vi "Measuring Complete Example (B).vi"() -> ()   [LabVIEW 2011]
uses:
  C:/Program Files/Metrohm Autolab/Autolab SDK 1.10/EcoChemie.Autolab.Sdk.dll
  EcoChemie.Autolab.Sdk.dll
panel:
  in  "Stop":bool
  out "PotentialApplied":dbl
  in  "Abort":bool
  in  "fileName":string
  out "IsMeasuring":bool
  in  "Save":bool
  in  "start measure":bool
  out "XY Graph":cluster{"Y":dbl[], "Y":dbl[]}[](graph)
  out "X: WE(1).Potential":dbl
  out "Y: WE(1).Current":dbl
  out "error out":errorcluster
  out "IsConnected":bool
  out "Y: EI_0.CalcCurrent":dbl[](array[numeric])
  out "X: SetpointApplied":dbl[](array[numeric])
  out "XY Graph 2":cluster{"Values":dbl[], "Values":dbl[]}(graph)
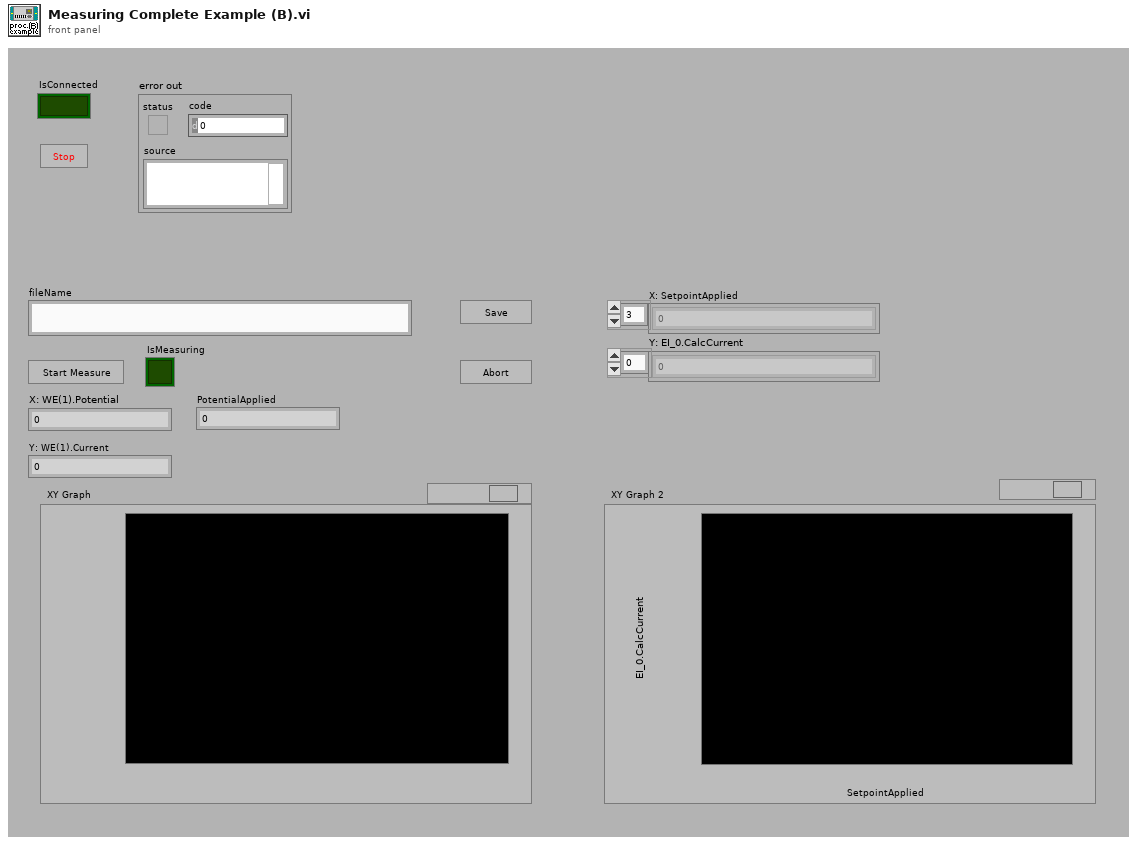
[diagram p1: front panel]
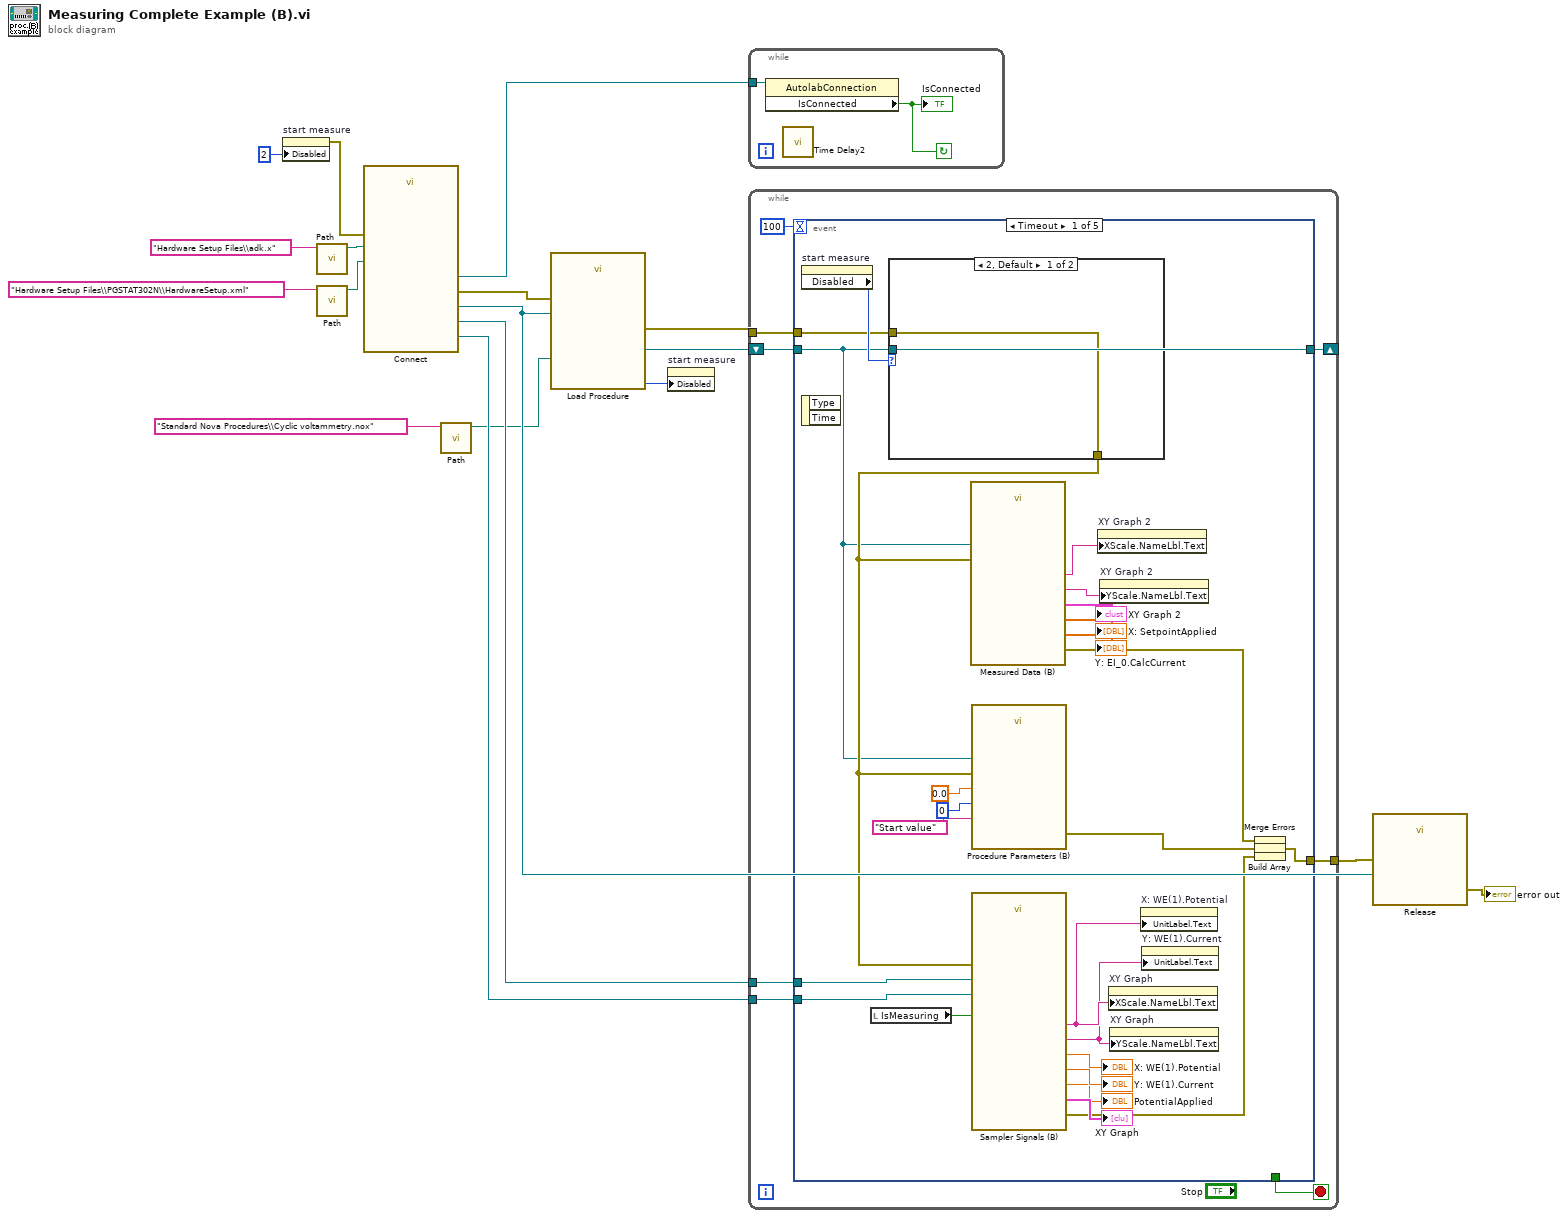
[diagram p0: block diagram]
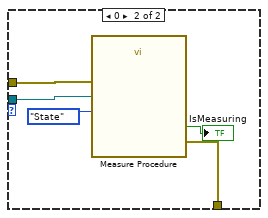
[diagram p2: hidden frame]
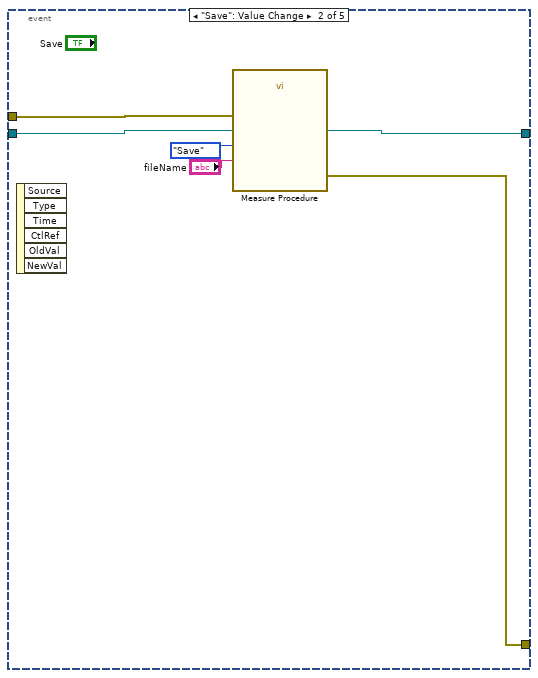
[diagram p3: hidden frame]
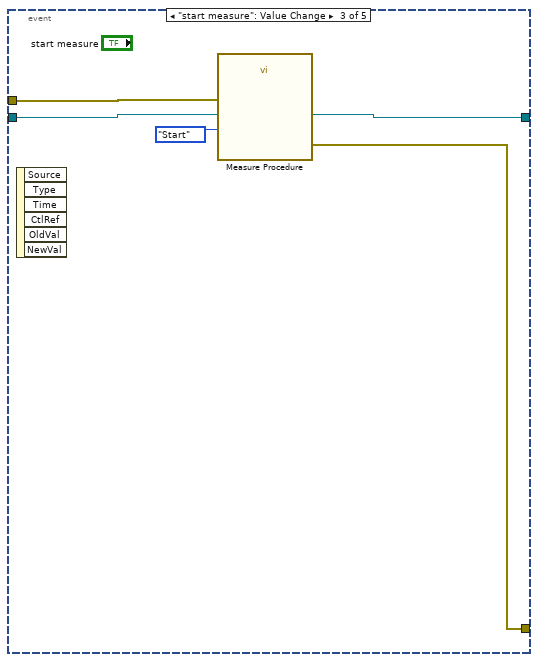
[diagram p4: hidden frame]
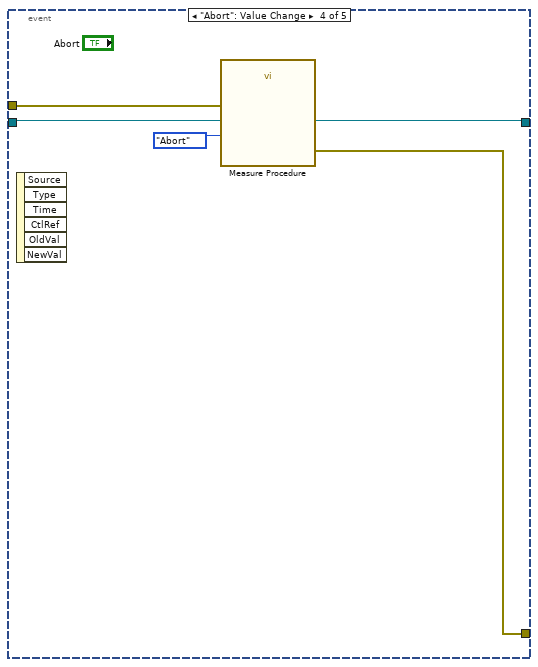
[diagram p5: hidden frame]
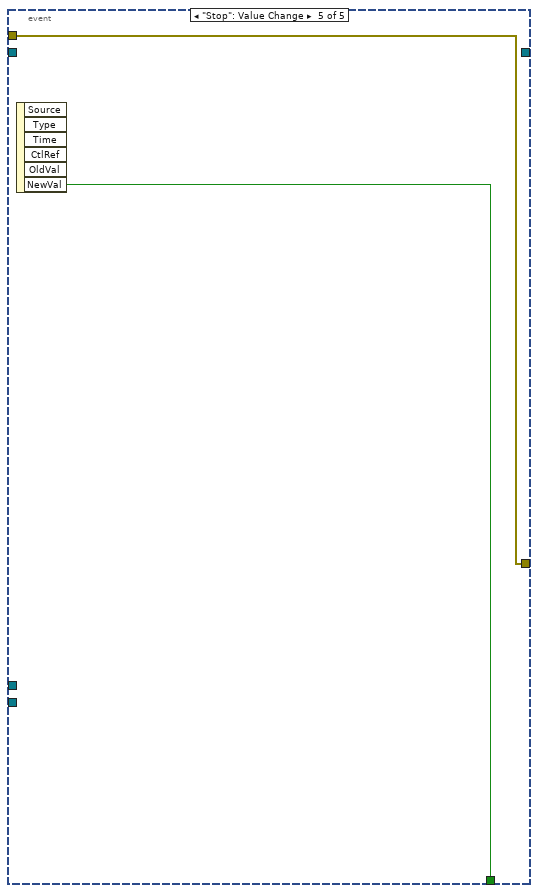
[diagram p6: hidden frame]
diagram:
  n1 = property on="start measure" class="Bool"("Disabled"=u8 2) -> (error out=w2:errorcluster)  [unwired: 2 in, 1 out]
  n2 = call "Path.vi"("name or relative path"="Hardware Setup Files\\adk.x") -> ("appended path"=w14:path)  [unwired: 10 in]
  n3 = call "Path.vi"("name or relative path"="Hardware Setup Files\\PGSTAT302N\\HardwareSetup.xml") -> ("appended path"=w11:path)  [unwired: 10 in]
  n4 = call "Connect.vi"("Embedded Exe File"=w14, "Hardware Setup File"=w11, "error in (no error)"=w2) -> ("Sampler"=w16:refnum<k24>, "AutolabConnection"=w17:refnum<k24>, "instrument"=w7:refnum<k24>, "Ei"=w15:refnum<k24>, "error out"=w8:errorcluster)  [unwired: 5 in, 3 out]
  n5 = call "Path.vi"("name or relative path"="Standard Nova Procedures\\Cyclic voltammetry.nox") -> ("appended path"=w4:path)  [unwired: 10 in]
  n6 = call "Load Procedure.vi"("error in (no error)"=w8, "Procedure"=w4, "Instrument"=w7) -> ("error out"=w6:errorcluster, "Numeric"=w3:i32, "LoadProcedure"=w5:refnum<k24>)  [unwired: 5 in, 1 out]
  n7 = property on="start measure" class="Bool"("Disabled"=w3) -> ()  [unwired: 2 in, 2 out]
  n8 = while {
    tunnel: w17 -> [w19]
    stop <- w20 continue-if-true
    n9 = property class="AutolabConnection"(reference=w19) -> ("IsConnected"=w20:bool)  [unwired: 1 in, 2 out]
    "IsConnected" <- w20
    n10 = call "Time Delay2"() -> ()  [unwired: 11 in, 1 out]
  }
  n11 = while {
    tunnel: w16 -> [w28]
    tunnel: w15 -> [w27]
    shift-right: [w25] -> _
    shift-left: w5 -> [w26]
    tunnel: w6 -> [w24]
    tunnel: [w22] -> w9
    stop <- w21 stop-if-true
    n12 = event shown="[0] Timeout" {
      selector: _ -> [_ _ _ _ _]
      dyn-events: _ -> [_ _ _ _ _]
      timeout: 100 -> [_ _ _ _ _]
      tunnel: w28 -> [w54 _ _ _ _]
      tunnel: w27 -> [w53 _ _ _ _]
      tunnel: w26 -> [w35 w61 w67 w71 _]
      tunnel: [w35 w61 w67 w71 _] -> w25
      tunnel: w24 -> [w34 w64 w68 w72 w74]
      tunnel: [w30 w62 w66 w70 w74] -> w22
      tunnel: [_ _ _ _ w75] -> w21
      event Timeout {
        n13 = property on="start measure" class="Bool"() -> ("Disabled"=w36:u8)  [unwired: 2 in, 2 out]
        n14 = event-data() -> ()  [unwired: 1 in, 2 out]
        n15 = local read "IsMeasuring"() -> (w44:bool)
        n16 = case shown="2, Default" w36 {
          tunnel: w35 -> [_ w58]
          tunnel: [w55 w57] -> w37
          tunnel: w34 -> [w55 w56]
          frame 2, Default {
          }
          frame 0 {
            n17 = call "Measure Procedure.vi"("error in"=w56, "Request for procedure"=enum16{"State", "Save", "Abort", "Start"}."State", "LoadProcedure"=w58) -> ("error out"=w57:errorcluster, "IsMeasuring"=→"IsMeasuring":bool)  [unwired: 7 in]
          }
        }
        n18 = call "Measured Data (B).vi"("LoadProcedure"=w35, "error in (no error)"=w37) -> ("Value X"=→"X: SetpointApplied":dbl[], "Value Y"=→"Y: EI_0.CalcCurrent":dbl[], "Signal X sel"=w49:string, "XY Graph"=→"XY Graph 2":cluster{"Values":dbl[], "Values":dbl[]}, "Signal Y sel"=w48:string, "error out"=w32:errorcluster)  [unwired: 12 in]
        n19 = call "Procedure Parameters (B).vi"("LoadProcedure"=w35, "Command Parameter"="Start value", "IntSet"=0, "DoubleSet"=0.0, "error in (no error)"=w37) -> ("error out"=w33:errorcluster)  [unwired: 10 in]
        n20 = call "Sampler Signals (B).vi"("Sampler"=w54, "EI"=w53, "measure"=w44, "error in"=w37) -> ("X"=→"X: WE(1).Potential":dbl, "Y"=→"Y: WE(1).Current":dbl, "Signal X"=w39:string, "XY Graph"=→"XY Graph":cluster{"Y":dbl[], "Y":dbl[]}[], "Signal Y"=w38:string, "PotentialApplied"=→"PotentialApplied":dbl, "error out"=w31:errorcluster)  [unwired: 5 in]
        n21 = property on="XY Graph 2" class="XYGraph (strict)"("XScale.NameLbl.Text"=w49) -> ()  [unwired: 2 in, 2 out]
        n22 = property on="XY Graph 2" class="XYGraph (strict)"("YScale.NameLbl.Text"=w48) -> ()  [unwired: 2 in, 2 out]
        n23 = property on="XY Graph" class="XYGraph (strict)"("XScale.NameLbl.Text"=w39) -> ()  [unwired: 2 in, 2 out]
        n24 = property on="XY Graph" class="XYGraph (strict)"("YScale.NameLbl.Text"=w38) -> ()  [unwired: 2 in, 2 out]
        n25 = property on="X: WE(1).Potential" class="DigNum (strict)"("UnitLabel.Text"=w39) -> ()  [unwired: 2 in, 2 out]
        n26 = property on="Y: WE(1).Current" class="DigNum (strict)"("UnitLabel.Text"=w38) -> ()  [unwired: 2 in, 2 out]
        n27 = Build Array(w32, w33, w31) -> (w29:errorcluster[])
        n28 = Merge Errors(w29) -> (w30:errorcluster)
      }
      event "Save": Value Change {
        n29 = event-data() -> ()  [unwired: 1 in, 6 out]
        n30 = call "Measure Procedure.vi"("error in"=w64, "fileName"="fileName", "Request for procedure"=enum16{"State", "Save", "Abort", "Start"}."Save", "LoadProcedure"=w61) -> ("error out"=w62:errorcluster)  [unwired: 6 in, 1 out]
      }
      event "start measure": Value Change {
        n31 = event-data() -> ()  [unwired: 1 in, 6 out]
        n32 = call "Measure Procedure.vi"("error in"=w68, "Request for procedure"=enum16{"State", "Save", "Abort", "Start"}."Start", "LoadProcedure"=w67) -> ("error out"=w66:errorcluster)  [unwired: 7 in, 1 out]
      }
      event "Abort": Value Change {
        n33 = event-data() -> ()  [unwired: 1 in, 6 out]
        n34 = call "Measure Procedure.vi"("error in"=w72, "Request for procedure"=enum16{"State", "Save", "Abort", "Start"}."Abort", "LoadProcedure"=w71) -> ("error out"=w70:errorcluster)  [unwired: 7 in, 1 out]
      }
      event "Stop": Value Change {
        n35 = event-data() -> ("NewVal"=w75:bool)  [unwired: 1 in, 5 out]
      }
    }
  }
  n36 = call "Release.vi"("error in (no error)"=w9, "Instrument"=w7) -> ("error out"=→"error out":errorcluster)  [unwired: 9 in]
